vi "WriteLabel.vi"(6 "TxPower":dbl, 7 "ATT":i32, 8 "error in (no error)":errorcluster, 9 "BW":string, 10 "Freq":i32, 11 "refnum out":refnum<file>) -> (0 "error out":errorcluster, 3 "refnum out 2":refnum<file>)   [LabVIEW 2012]
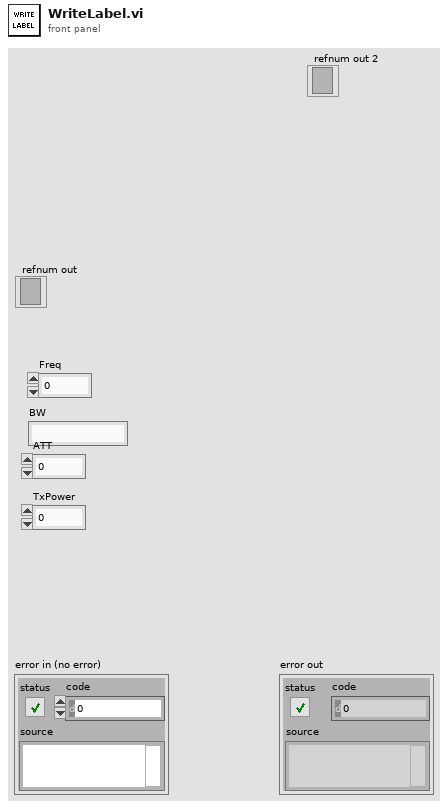
[diagram p1: front panel]
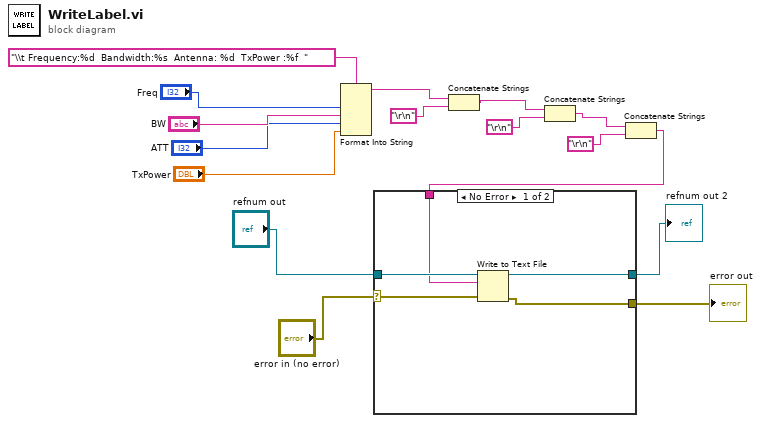
[diagram p0: block diagram]
diagram:
  n1 = Format Into String(format string="\\t Frequency:%d  Bandwidth:%s  Antenna: %d  TxPower :%f  ", "Freq", "BW", "ATT", "TxPower") -> (resulting string=w7:string)  [unwired: 2 in, 1 out]
  n2 = Concatenate Strings(w7, "\r\n") -> (w4:string)
  n3 = Concatenate Strings(w4, "\r\n") -> (w2:string)
  n4 = Concatenate Strings(w2, "\r\n") -> (w1:string)
  n5 = case shown="No Error" "error in (no error)" {
    selector: "error in (no error)" -> [w20 w22]
    tunnel: [w19 w22] -> w15
    tunnel: "refnum out" -> [w21 _]
    tunnel: w1 -> [w18 _]
    tunnel: [w17 _] -> w8
    frame No Error {
      n6 = Write to Text File(file (use dialog)=w21, text=w18, error in=w20) -> (refnum out=w17:refnum<file>, error out=w19:errorcluster)  [unwired: 1 in, 1 out]
    }
    frame Error {
    }
  }
  "error out" <- w15
  "refnum out 2" <- w8
